vi "Get Header Info.vi"(11 "XML in":refnum<class "XML.lvclass">) -> (0 "Meta Data":string, 1 "Attribute Type":string, 2 "Global":string, 3 "XML out":refnum<class "XML.lvclass">, 4 "Tag Name":string, 5 "GUID":string, 6 "Attribute Name":string)   [LabVIEW 2020, in "XML.lvlib" / "XML.lvclass"]
uses:
  <vilib>/gpm_packages/@cs/persistence/source/XML/XML.lvclass
  <vilib>/gpm_packages/@cs/persistence/source/XML/XML.lvclass/XML.ctl
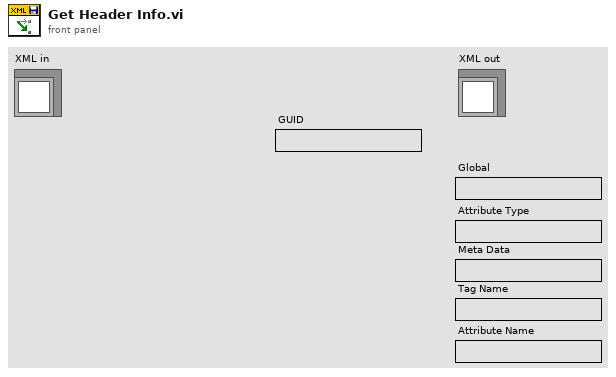
[diagram p1: front panel]
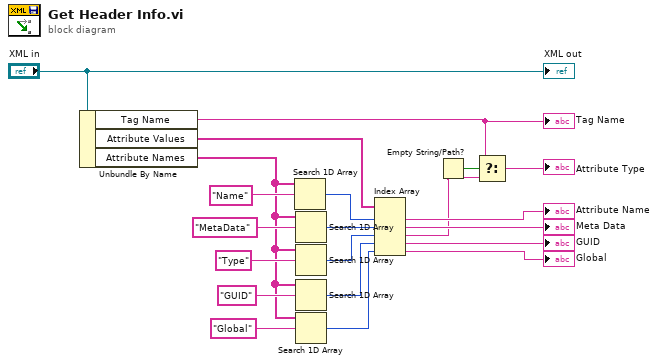
[diagram p0: block diagram]
diagram:
  n1 = Unbundle By Name("XML in") -> ("Tag Name"=w3:string, "Attribute Values"=w2:string[], "Attribute Names"=w1:string[])
  "Tag Name" <- w3
  n2 = Search 1D Array(1D array=w1, element="Name") -> (index of element=w20:i32)  [unwired: 1 in]
  n3 = Search 1D Array(1D array=w1, element="MetaData") -> (index of element=w16:i32)  [unwired: 1 in]
  n4 = Search 1D Array(1D array=w1, element="Type") -> (index of element=w18:i32)  [unwired: 1 in]
  n5 = Search 1D Array(1D array=w1, element="GUID") -> (index of element=w8:i32)  [unwired: 1 in]
  n6 = Search 1D Array(1D array=w1, element="Global") -> (index of element=w5:i32)  [unwired: 1 in]
  n7 = Index Array(array=w2, index #1=w20, index #2=w16, index #3=w18, index #4=w8, index #5=w5) -> (element #1=→"Attribute Name":string, element #2=→"Meta Data":string, element #3=w11:string, element #4=→"GUID":string, element #5=→"Global":string)
  n8 = Empty String/Path?(string/path=w11) -> (empty?=w12:bool)
  n9 = Select(t=w3, s=w12, f=w11) -> (s? t:f=→"Attribute Type":string)
  "XML out" <- "XML in"
